vi "Conf Scaling.vi"(0 "VISA Resource Name":refnum<visa-resource-name>, 1 "Enable Scaling? (T:Enable)":bool=TRUE, 2 "Set/Check (F:Set)":bool, 5 "Gain (1)":dbl=1.0 min=-1000000000000.0 max=1000000000000.0 format="%.2f", 7 "Offset (0)":dbl min=-1000000000000.0 max=1000000000000.0 format="%.2f", 9 "Units (empty)":string, 11 "error in (no error)":errorcluster, 12 "Check (0:Gain)":enum16{"Gain", "Offset", "Status", "Units"}(ring), 13 "Channel List (empty)":string) -> (4 "VISA Resource Name Out":refnum<visa-resource-name>, 8 "Configuration?":string, 15 "error out":errorcluster)   [LabVIEW 2020, in "Agilent 34970.lvlib"]
doc: "This VI allows you to control or check measurement scaling and units. For example, you can add a gain and offset to certain channels' readings. You can also add a custom unit label."
uses:
  Agilent 34970.lvlib
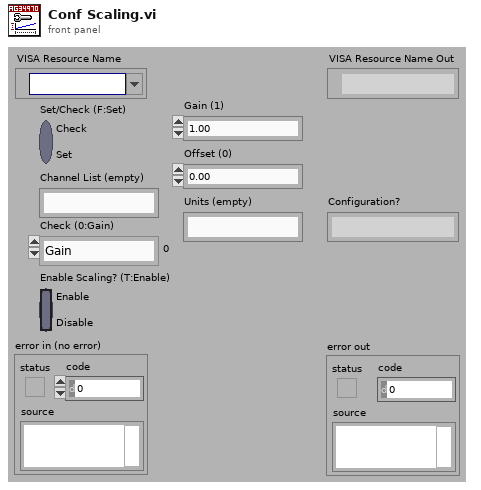
[diagram p1: front panel]
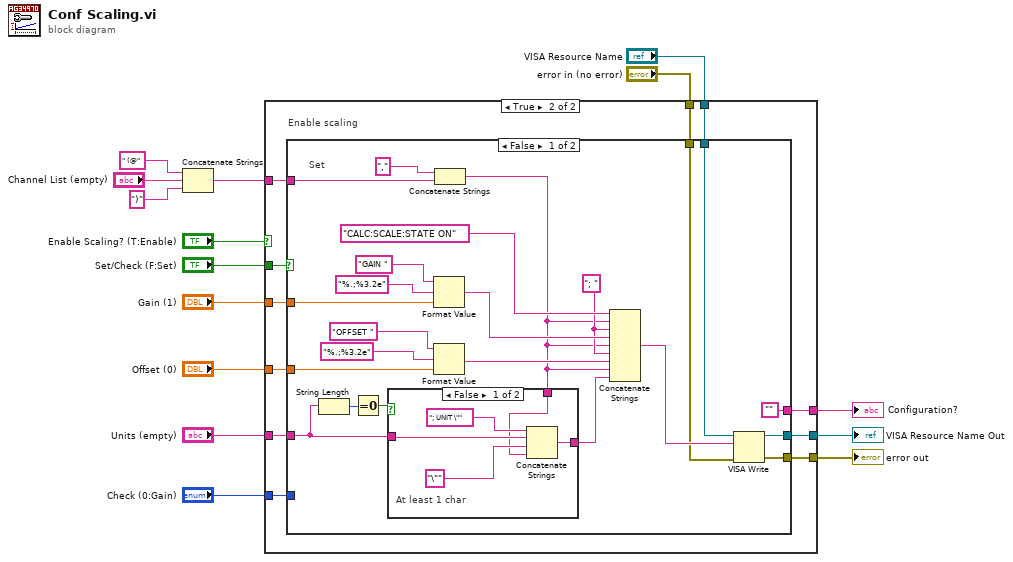
[diagram p0: block diagram]
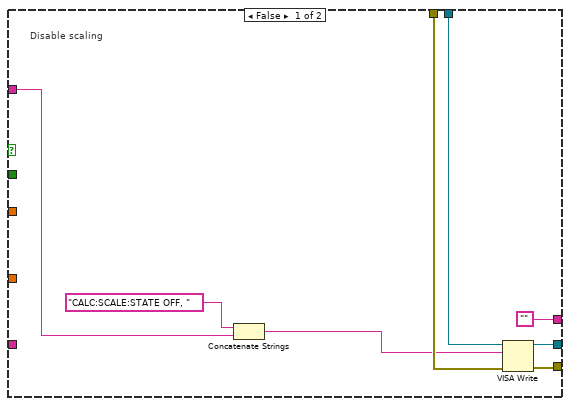
[diagram p2: hidden frame]
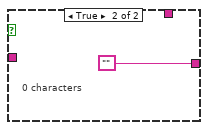
[diagram p3: hidden frame]
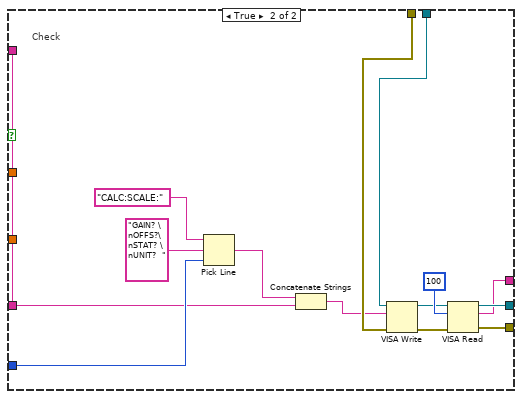
[diagram p4: hidden frame]
diagram:
  n1 = Concatenate Strings(" (@", "Channel List (empty)", ")") -> (w12:string)
  n2 = case shown="True" "Enable Scaling? (T:Enable)" {
    tunnel: w12 -> [w16 w33]
    tunnel: "Check (0:Gain)" -> [_ w29]
    tunnel: "Set/Check (F:Set)" -> [_ w34]
    tunnel: "Gain (1)" -> [_ w32]
    tunnel: "Offset (0)" -> [_ w31]
    tunnel: "Units (empty)" -> [_ w30]
    tunnel: "error in (no error)" -> [w19 w28]
    tunnel: "VISA Resource Name" -> [w18 w27]
    tunnel: [w21 w26] -> w2
    tunnel: [w22 w25] -> w1
    tunnel: ["" w24] -> w5
    frame False {
      # "Disable scaling"
      n3 = Concatenate Strings("CALC:SCALE:STATE OFF, ", w16) -> (w17:string)
      n4 = VISA Write(VISA resource name=w18, write buffer=w17, error in (no error)=w19) -> (VISA resource name out=w21:refnum<visa-resource-name>, error out=w22:errorcluster)  [unwired: 1 out]
    }
    frame True {
      # "Enable scaling"
      n5 = case shown="False" w34 {
        tunnel: w33 -> [w56 w74]
        tunnel: w32 -> [w55 _]
        tunnel: w31 -> [w50 _]
        tunnel: w30 -> [w35 _]
        tunnel: w29 -> [_ w75]
        tunnel: w28 -> [w36 w69]
        tunnel: w27 -> [w46 w64]
        tunnel: [w45 w68] -> w26
        tunnel: [w44 w67] -> w25
        tunnel: ["" w66] -> w24
        frame False {
          w40 = "; "
          # "Set"
          n6 = String Length(string=w35) -> (length=w42:i32)
          n7 = Equal To 0?(x=w42) -> (x = 0?=w41:bool)
          n8 = Format Value(string ("")="GAIN ", format string="%.;%3.2e", value (0)=w55) -> (output string=w48:string)
          n9 = Format Value(string ("")="OFFSET ", format string="%.;%3.2e", value (0)=w50) -> (output string=w47:string)
          n10 = Concatenate Strings(",", w56) -> (w39:string)
          n11 = case shown="False" w41 {
            tunnel: w35 -> [w60 _]
            tunnel: [w61 ""] -> w38
            tunnel: w39 -> [w58 _]
            frame False {
              # "At least 1 char"
              n12 = Concatenate Strings("; UNIT \"", w60, "\"", w58) -> (w61:string)
            }
            frame True {
              # "0 characters"
            }
          }
          n13 = Concatenate Strings("CALC:SCALE:STATE ON", w39, w40, w48, w39, w40, w47, w39, w38) -> (w37:string)
          n14 = VISA Write(VISA resource name=w46, write buffer=w37, error in (no error)=w36) -> (VISA resource name out=w45:refnum<visa-resource-name>, error out=w44:errorcluster)  [unwired: 1 out]
        }
        frame True {
          # "Check"
          n15 = Pick Line(string ("")="CALC:SCALE:", multi-line string="GAIN? \nOFFS?\nSTAT? \nUNIT?  ", line index=w75) -> (output string=w73:string)
          n16 = Concatenate Strings(w73, w74) -> (w65:string)
          n17 = VISA Write(VISA resource name=w64, write buffer=w65, error in (no error)=w69) -> (VISA resource name out=w71:refnum<visa-resource-name>, error out=w70:errorcluster)  [unwired: 1 out]
          n18 = VISA Read(VISA resource name=w71, byte count=u32 100 ("byte count (0)"), error in (no error)=w70) -> (VISA resource name out=w68:refnum<visa-resource-name>, read buffer=w66:string, error out=w67:errorcluster)  [unwired: 1 out]
        }
      }
    }
  }
  "Configuration?" <- w5
  "VISA Resource Name Out" <- w2
  "error out" <- w1
